vi "Analog Replays Page.vi"(8 "error in (no error)":errorcluster, 11 "Node Ptr":T1 format="%.0x") -> (0 "error out":errorcluster)   [LabVIEW 2019, in "Engine Simulation Toolkit System Explorer.lvlib"]
uses:
  Engine Simulation Toolkit System Explorer.lvlib
  <vilib>/NI VeriStand/Custom Device API/Custom Device Item Ref.ctl
  Shared/Properties.vi
  Shared/Constants and GUIDs.vi
  <vilib>/NI VeriStand/Custom Device API/Custom Device API.lvlib
  Shared/Engine Simulation Toolkit Shared.lvlib
  <vilib>/NI VeriStand/Custom Device Tools/Custom Device Utility Library/Custom Device Utility Library.lvlib
panel:
  in  "remove":bool
  in  "add":bool
  in  "Replay listbox":i32[](listbox) caption="Available Analog Replays"
  in  "Header":cluster{"Section Name":string}={"Section Name"="Analog Replays Settings"}
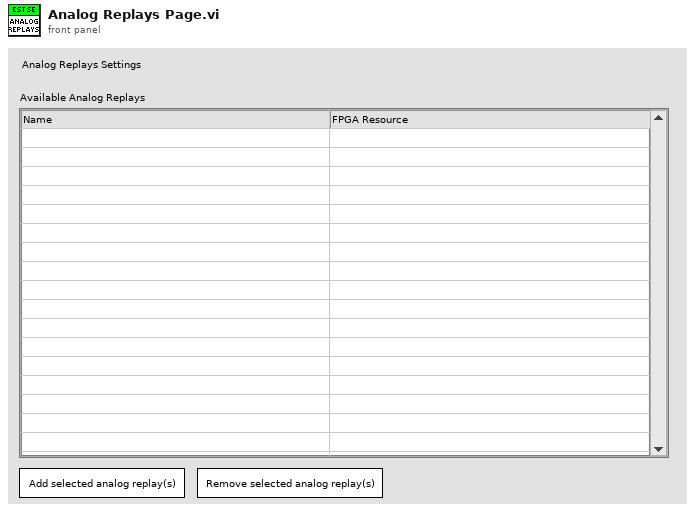
[diagram p1: front panel]
types:
  T1 = typedef "Custom Device API.lvlib/Custom Device Item Ref.ctl" = u64
  T2 = enum8{"Enabled", "Disabled", "Disabled and Grayed Out"}
  T3 = cluster{"ip list property name":string, string[]}[]
  T4 = typedef "Custom Device API.lvlib/Custom Device Commands.ctl" = enum16{"Default", "Item renamed", "Shutdown", "Dynamic button pressed"}
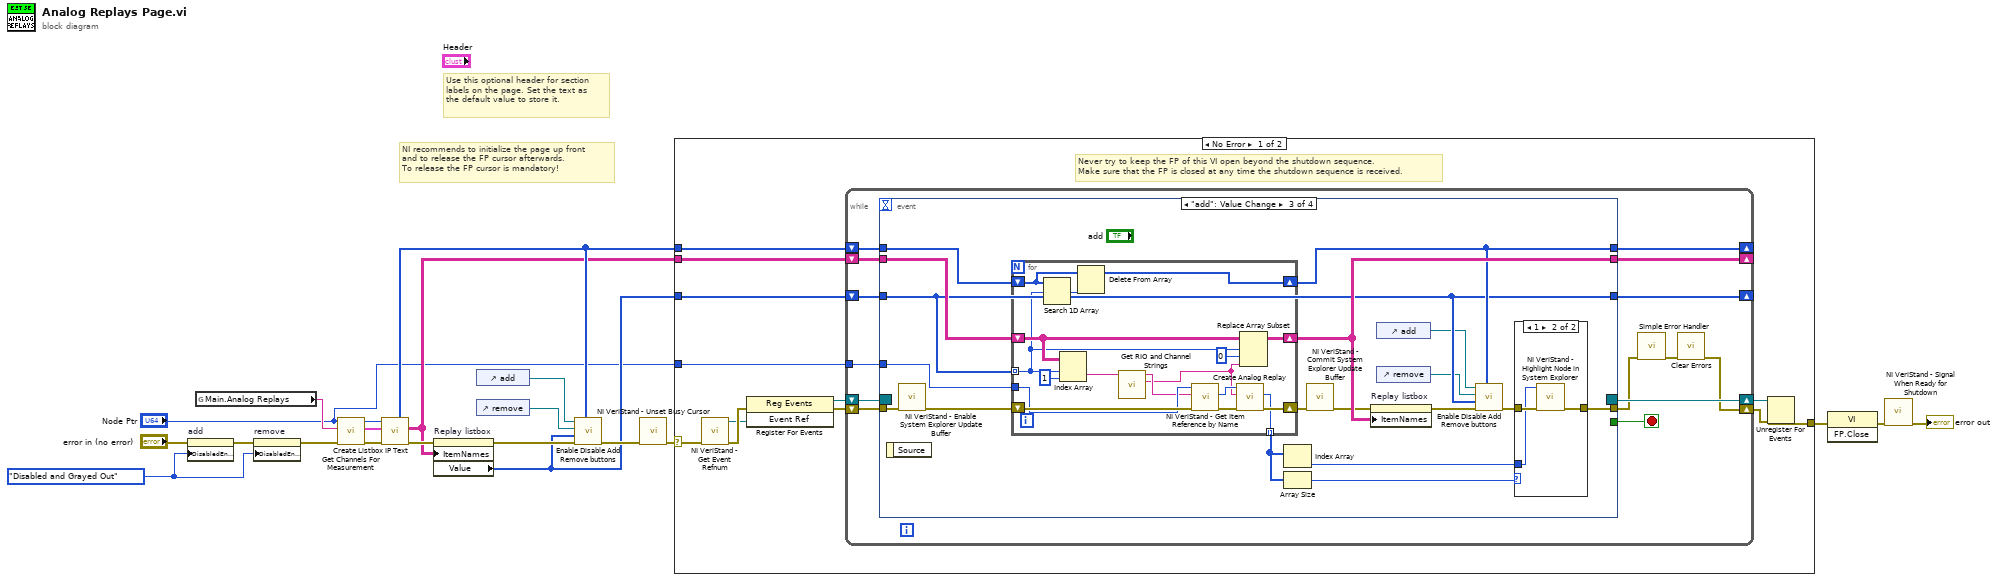
[diagram p0: block diagram]
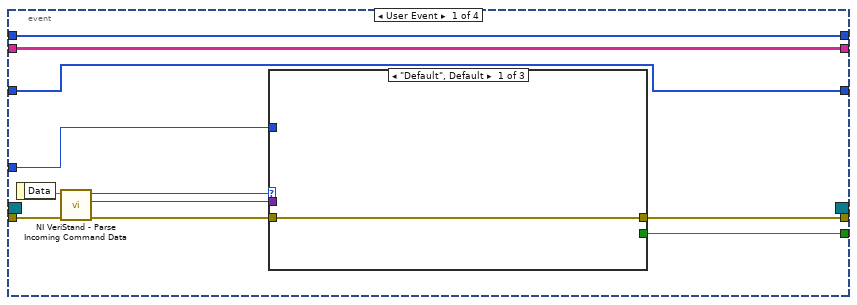
[diagram p2: hidden frame]
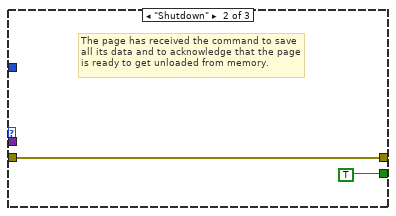
[diagram p3: hidden frame]
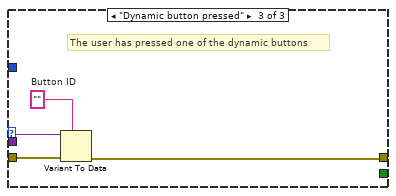
[diagram p4: hidden frame]
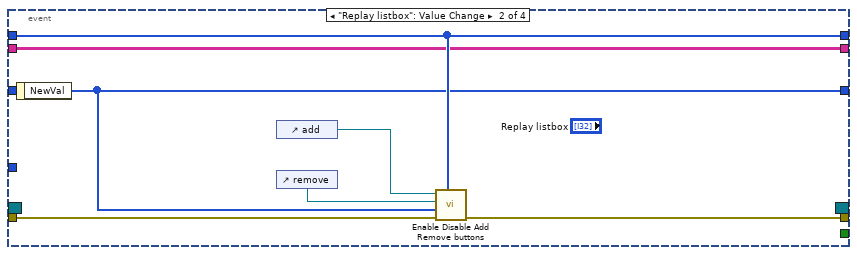
[diagram p5: hidden frame]
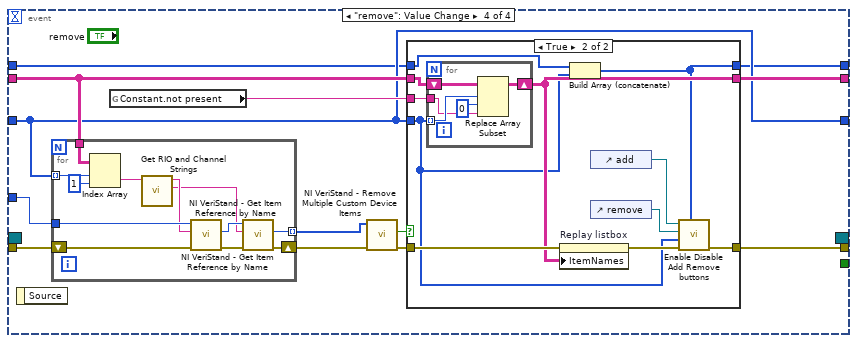
[diagram p7: hidden frame]
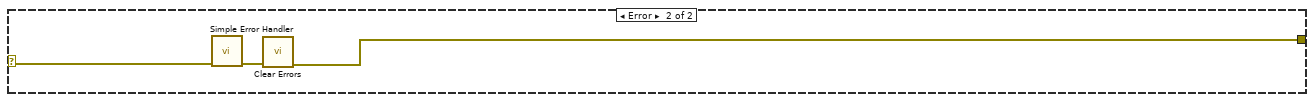
[diagram p9: hidden frame]
diagram:
  w13 = T2."Disabled and Grayed Out" ("Disabled")
  # "Use this optional header for section labels on the page. Set the text as the default value to store it."
  # "NI recommends to initialize the page up front\nand to release the FP cursor afterwards.\nTo release the FP cursor is mandatory!"
  n1 = property on="add" class="Bool"(error in="error in (no error)", "DisabledEnum"=w13) -> (error out=w14:errorcluster)  [unwired: 1 in, 1 out]
  n2 = global read "Properties.vi" "Main.Analog Replays"() -> (w4:string)
  n3 = property on="remove" class="Bool"(error in=w14, "DisabledEnum"=w13) -> (error out=w5:errorcluster)  [unwired: 1 in, 1 out]
  n4 = call "Get Channels For Measurement.vi"("error in (no error)"=w5, "property name"=w4, "Node Ptr in"="Node Ptr") -> ("error out"=w17:errorcluster, "rios and channels"=w1:T3, "Node Ptr out"=w2:T1)  [unwired: 6 in]
  n5 = call "Create Listbox IP Text.vi"("error in (no error)"=w17, "rios and analog replays"=w1, "Section Ref in"=w2) -> ("error out"=w15:errorcluster, "listbox text"=w6:string[][], "not present item indexes"=w8:i32[])  [unwired: 5 in, 1 out]
  n6 = property on="Replay listbox" class="MCListbox (strict)"(error in=w15, "ItemNames"=w6) -> (error out=w10:errorcluster, "Value"=w7:i32[])  [unwired: 1 in, 1 out]
  n7 = control-ref of="add"() -> (w11:refnum<vi>)
  n8 = control-ref of="remove"() -> (w12:refnum<vi>)
  n9 = call "Enable Disable Add Remove buttons.vi"("not present item indexes"=w8, "error in (no error)"=w10, "selected items"=w7, "remove button"=w12, "add button"=w11) -> ("error out"=w9:errorcluster)  [unwired: 6 in]
  n10 = call <vilib>:"NI VeriStand - Unset Busy Cursor.vi"("error in (no error)"=w9) -> ("error out"=w18:errorcluster)  [unwired: 10 out]
  n11 = case shown="No Error" w18 {
    selector: w18 -> [w25 w158]
    tunnel: [w30 w156] -> w21
    tunnel: "Node Ptr" -> [w26 _]
    tunnel: w6 -> [w24 _]
    tunnel: w8 -> [w23 _]
    tunnel: w7 -> [w22 _]
    frame No Error {
      # "Never try to keep the FP of this VI open beyond the shutdown sequence.\nMake sure that the FP is closed at any time the shutdown sequence is received."
      n12 = call <vilib>:"NI VeriStand - Get Event Refnum.vi"("error in (no error)"=w25) -> ("error out"=w33:errorcluster, "Event Ref"=w29:refnum<user-event>)  [unwired: 9 out]
      n13 = register-events(error in=w33, w29) -> (reference out=w27:refnum<event-registration>, error out=w28:errorcluster)  [unwired: 1 in]
      n14 = while {
        tunnel: w26 -> [w43]
        shift-right: [w40] -> w31
        shift-left: w28 -> [w46]
        shift-right: [w47] -> w32
        shift-left: w27 -> [w45]
        shift-right: [w38] -> _
        shift-left: w22 -> [w35]
        shift-right: [w36] -> _
        shift-left: w23 -> [w34]
        shift-right: [w37] -> _
        shift-left: w24 -> [w39]
        stop <- w44 stop-if-true
        n15 = event shown="[2] \"add\": Value Change" {
          selector: w45 -> [_ _ _ _]
          dyn-events: [_ _ _ _] -> w47
          timeout: _ -> [_ _ _ _]
          tunnel: w46 -> [w58 w72 w90 w123]
          tunnel: [w54 _ _ _] -> w44
          tunnel: [w53 w71 w75 w124] -> w42
          tunnel: w43 -> [w52 _ w89 w122]
          tunnel: w39 -> [w49 w66 w88 w117]
          tunnel: w34 -> [w48 w68 w87 w113]
          tunnel: [w50 w67 w82 w114] -> w38
          tunnel: w35 -> [w50 _ w82 w114]
          tunnel: [w49 w66 w85 w115] -> w37
          tunnel: [w48 w68 w83 w112] -> w36
          event User Event {
            n16 = event-data() -> ("Data"=w57:string)  [unwired: 1 out]
            n17 = call <vilib>:"NI VeriStand - Parse Incoming Command Data.vi"("error in (no error)"=w58, "Incoming data"=w57) -> ("error out"=w56:errorcluster, "Outgoing data"=w51:variant, "Action"=w55:T4)  [unwired: 7 out]
            n18 = case shown="\"Default\", Default" w55 {
              tunnel: w56 -> [w59 w60 w65]
              tunnel: [_ TRUE _] -> w54
              tunnel: [w59 w60 w62] -> w53
              tunnel: w52 -> [_ _ _]
              tunnel: w51 -> [_ _ w64]
              frame "Default", Default {
              }
              frame "Shutdown" {
                # "The page has received the command to save all its data and to acknowledge that the page is ready to get unloaded from memory."
              }
              frame "Dynamic button pressed" {
                w63 = ""  # Button ID
                # "The user has pressed one of the dynamic buttons"
                n19 = Variant To Data(error in=w65, type=w63, Variant=w64) -> (error out=w62:errorcluster)  [unwired: 1 out]
              }
            }
          }
          event "Replay listbox": Value Change {
            n20 = event-data() -> ("NewVal"=w67:i32[])  [unwired: 1 out]
            n21 = control-ref of="add"() -> (w70:refnum<vi>)
            n22 = control-ref of="remove"() -> (w69:refnum<vi>)
            n23 = call "Enable Disable Add Remove buttons.vi"("not present item indexes"=w68, "error in (no error)"=w72, "selected items"=w67, "remove button"=w69, "add button"=w70) -> ("error out"=w71:errorcluster)  [unwired: 6 in]
          }
          event "add": Value Change {
            n24 = event-data() -> ()  [unwired: 2 out]
            n25 = call <vilib>:"NI VeriStand - Enable System Explorer Update Buffer.vi"("error in (no error)"=w90) -> ("error out"=w78:errorcluster)  [unwired: 10 in]
            n26 = for {
              tunnel: w89 -> [w99]
              shift-right: [w111] -> w86
              shift-left: w78 -> [w101]
              tunnel: w82 -> [w106] mode=indexing
              shift-right: [w108] -> w85
              shift-left: w88 -> [w109]
              shift-right: [w103] -> w83
              shift-left: w87 -> [w105]
              tunnel: [w102] -> w77 mode=indexing
              n27 = Search 1D Array(1D array=w105, element=w106) -> (index of element=w104:i32)  [unwired: 1 in]
              n28 = Index Array(array=w109, index (row)=w106, index (col)=1 ("disabled index (col)")) -> (element=w95:string)
              n29 = Delete From Array(array=w105, index=w104) -> (array with subset deleted=w103:i32[])  [unwired: 1 in, 1 out]
              n30 = call "Get RIO and Channel Strings.vi"("rio/channel"=w95) -> ("channel"=w96:string, "rio"=w97:string)  [unwired: 9 in]
              n31 = call <vilib>:"NI VeriStand - Get Item Reference by Name.vi"("error in (no error)"=w101, "Item Name"=w97, "Parent Ref in"=w99) -> ("error out"=w100:errorcluster, "Item Ref"=w98:T1)  [unwired: 5 in, 2 out]
              n32 = call "Create Analog Replay.vi"("error in (no error)"=w100, "analog replay name"=w96, "Section Ptr"=w98) -> ("error out"=w111:errorcluster, "Analog replay ref"=w102:T1)  [unwired: 6 in, 1 out]
              n33 = Replace Array Subset(array=w109, new element=w96, index (row)=w106, index (col)=0 ("disabled index (col)")) -> (w108:string[][])
            }
            n34 = Index Array(array=w77) -> (element=w73:T1)  [unwired: 1 in]
            n35 = Array Size(array=w77) -> (size(s)=w76:i32)
            n36 = call <vilib>:"NI VeriStand - Commit System Explorer Update Buffer.vi"("error in (no error)"=w86) -> ("error out"=w79:errorcluster)  [unwired: 10 in]
            n37 = property on="Replay listbox" class="MCListbox (strict)"(error in=w79, "ItemNames"=w85) -> (error out=w84:errorcluster)  [unwired: 1 in, 1 out]
            n38 = control-ref of="add"() -> (w81:refnum<vi>)
            n39 = control-ref of="remove"() -> (w80:refnum<vi>)
            n40 = call "Enable Disable Add Remove buttons.vi"("not present item indexes"=w83, "error in (no error)"=w84, "selected items"=w82, "remove button"=w80, "add button"=w81) -> ("error out"=w74:errorcluster)  [unwired: 6 in]
            n41 = case shown="1" w76 {
              tunnel: [w91 w93] -> w75
              tunnel: w74 -> [w91 w94]
              tunnel: w73 -> [_ w92]
              frame Default {
              }
              frame 1 {
                n42 = call <vilib>:"NI VeriStand - Highlight Node in System Explorer.vi"("error in (no error)"=w94, "Item Ref in"=w92) -> ("error out"=w93:errorcluster)  [unwired: 8 in, 1 out]
              }
            }
          }
          event "remove": Value Change {
            n43 = event-data() -> ()  [unwired: 2 out]
            n44 = for {
              tunnel: w114 -> [w154] mode=indexing
              tunnel: w117 -> [w155]
              tunnel: w122 -> [w152]
              tunnel: [w146] -> w120 mode=indexing
              shift-right: [w147] -> w121
              shift-left: w123 -> [w153]
              n45 = Index Array(array=w155, index (row)=w154, index (col)=1 ("disabled index (col)")) -> (element=w150:string)
              n46 = call "Get RIO and Channel Strings.vi"("rio/channel"=w150) -> ("channel"=w144:string, "rio"=w149:string)  [unwired: 9 in]
              n47 = call <vilib>:"NI VeriStand - Get Item Reference by Name.vi"("error in (no error)"=w153, "Item Name"=w149, "Parent Ref in"=w152) -> ("error out"=w148:errorcluster, "Item Ref"=w145:T1)  [unwired: 5 in, 2 out]
              n48 = call <vilib>:"NI VeriStand - Get Item Reference by Name.vi"("error in (no error)"=w148, "Item Name"=w144, "Parent Ref in"=w145) -> ("error out"=w147:errorcluster, "Item Ref"=w146:T1)  [unwired: 5 in, 2 out]
            }
            n49 = global read "Constants and GUIDs.vi" "Constant.not present"() -> (w116:string)
            n50 = call <vilib>:"NI VeriStand - Remove Multiple Custom Device Items.vi"("error in (no error)"=w121, "Item Refs in"=w120) -> ("error out"=w119:errorcluster, "Deleted?"=w118:bool)  [unwired: 8 in]
            n51 = case shown="True" w118 {
              tunnel: [w126 w137] -> w124
              tunnel: w119 -> [w126 w134]
              tunnel: w114 -> [_ w129]
              tunnel: w117 -> [w127 w133]
              tunnel: w116 -> [_ w132]
              tunnel: [w127 w131] -> w115
              tunnel: w113 -> [w125 w130]
              tunnel: [w125 w128] -> w112
              frame False {
              }
              frame True {
                n52 = for {
                  tunnel: w129 -> [w141] mode=indexing
                  shift-right: [w142] -> w131
                  shift-left: w133 -> [w143]
                  tunnel: w132 -> [w139]
                  n53 = Replace Array Subset(array=w143, new element=w139, index (row)=w141, index (col)=0 ("disabled index (col)")) -> (w142:string[][])
                }
                n54 = property on="Replay listbox" class="MCListbox (strict)"(error in=w134, "ItemNames"=w131) -> (error out=w138:errorcluster)  [unwired: 1 in, 1 out]
                n55 = Build Array (concatenate)(w130, w129) -> (w128:i32[])
                n56 = control-ref of="add"() -> (w136:refnum<vi>)
                n57 = control-ref of="remove"() -> (w135:refnum<vi>)
                n58 = call "Enable Disable Add Remove buttons.vi"("not present item indexes"=w128, "error in (no error)"=w138, "selected items"=w129, "remove button"=w135, "add button"=w136) -> ("error out"=w137:errorcluster)  [unwired: 6 in]
              }
            }
          }
        }
        n59 = call <vilib>:"Simple Error Handler.vi"("error in (no error)"=w42) -> ("error out"=w41:errorcluster)  [unwired: 1 in, 7 out]
        n60 = call <vilib>:"Clear Errors.vi"("error in (no error)"=w41) -> ("error out"=w40:errorcluster)  [unwired: 1 in, 5 out]
      }
      n61 = Unregister For Events(event registration refnum=w32, error in=w31) -> (error out=w30:errorcluster)
    }
    frame Error {
      n62 = call <vilib>:"Simple Error Handler.vi"("error in (no error)"=w158) -> ("error out"=w157:errorcluster)  [unwired: 1 in, 7 out]
      n63 = call <vilib>:"Clear Errors.vi"("error in (no error)"=w157) -> ("error out"=w156:errorcluster)  [unwired: 1 in, 5 out]
    }
  }
  n64 = invoke class="VI" method="FP.Close"(error in=w21) -> (error out=w20:errorcluster)  [unwired: 2 in, 2 out]
  n65 = call <vilib>:"NI VeriStand - Signal When Ready for Shutdown.vi"("error in (no error)"=w20) -> ("error out"=→"error out":errorcluster)  [unwired: 10 out]
